vi "String2Pointer.vi"(8 "error in (no error)":errorcluster, 11 "SQL Statement":string) -> (0 "error out":errorcluster, 2 "size":i32, 3 "pointer":i64)   [LabVIEW 2019, in "SQLiteConnection.lvclass"]
uses:
  SQLiteConnection.lvclass
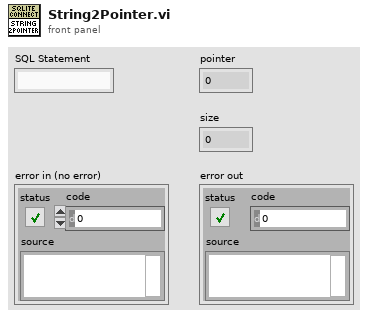
[diagram p1: front panel]
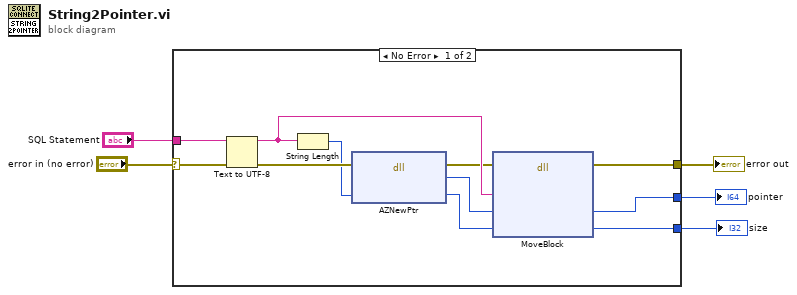
[diagram p0: block diagram]
diagram:
  n1 = case shown="No Error" "error in (no error)" {
    selector: "error in (no error)" -> [w6 w17]
    tunnel: "SQL Statement" -> [w15 _]
    tunnel: [w14 _] -> w4
    tunnel: [w13 _] -> w3
    tunnel: [w12 w17] -> w2
    frame No Error {
      n2 = Text to UTF-8(8:w6, 11:w15) -> (0:w11:errorcluster, 3:w16:string)  [unwired: 1 in]
      n3 = String Length(string=w16) -> (length=w7:i32)
      n4 = dll-call lib="LabVIEW" fn="AZNewPtr"(error in=w11, "size"=w7) -> (error out=w8:errorcluster, "pointer"=w10:i64, "size"=w9:i32)  [unwired: 2 in, 1 out]
      n5 = dll-call lib="LabVIEW" fn="MoveBlock"(error in=w8, "string"=w16, "pointer"=w10, "size"=w9) -> (error out=w12:errorcluster, "pointer"=w13:i64, "size"=w14:i32)  [unwired: 4 in, 1 out]
    }
    frame Error {
    }
  }
  "size" <- w4
  "pointer" <- w3
  "error out" <- w2
